vi "102_EON_presence_absence.vi"(8 "error in (no error)":errorcluster, 10 "Measurement ROI":T1 {"Contours"."Type" items=["No Selection", "Point", "Line", "Rectangle", "Oval", "Polygon", "Freehand Region", "Annulus", "Unused2", "Unused3", "Broken Line", "Freehand Line", "Rotated Rectangle"]}, 11 "Image In":T2(plugin-control)) -> (0 "error out":errorcluster, 2 "EON Presence/Absence":bool, 3 "Blob Center":cluster{"Center X":dbl, "Center Y":dbl})   [LabVIEW 2015]
uses:
  <vilib>/vision/NI_Vision_Development_Module.lvlib
  FrameworkOverrides/Algorithm.lvclass
panel:
  out "Area":dbl[](array[numeric])
  out "Area":dbl
  out "Y Coord":dbl[](array[numeric])
  out "Number of Particles":i32
  out "subarray 2":dbl[](array[numeric])
  out "index of element":i32
  out "Array":bool[](array[boolean])
  out "X Coord":dbl[](array[numeric])
  out "Image 2":T2(plugin-control)
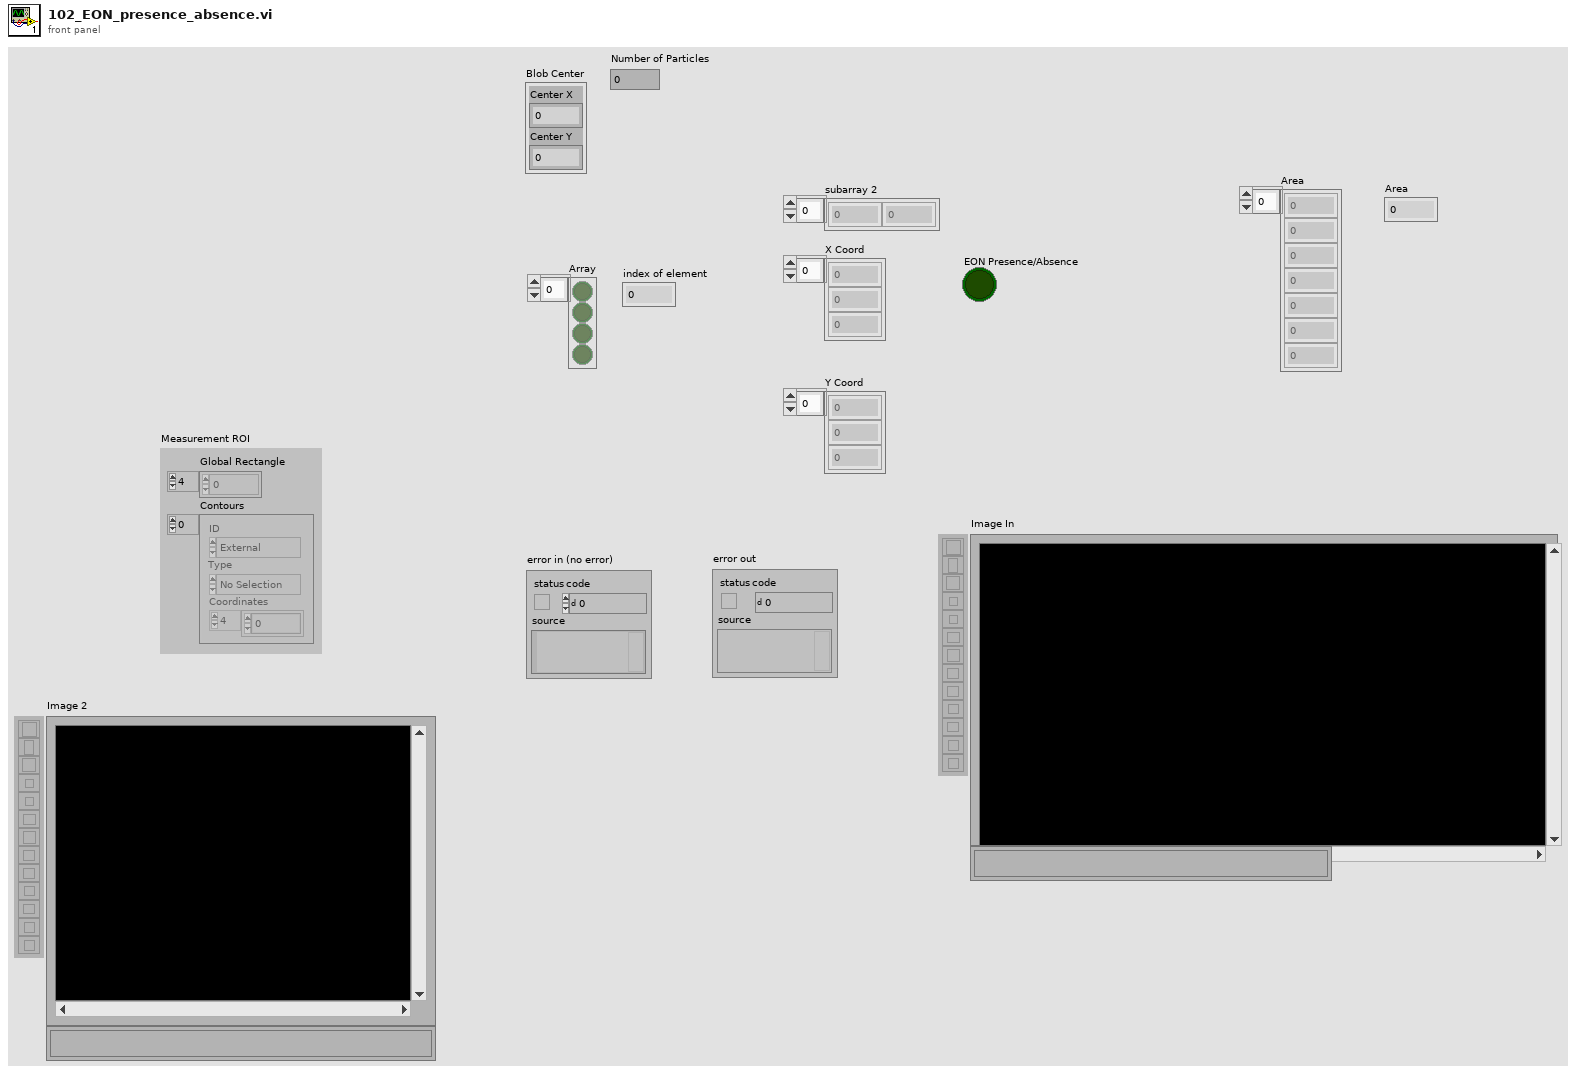
[diagram p1: front panel]
types:
  T1 = typedef "ROI Descriptor" = cluster{"Global Rectangle":i32[], "Contours":cluster{"ID":enum32{"External", "Internal"}, "Type":u32, "Coordinates":i32[]}[]}
  T2 = typedef "IMAQ Image.ctl" = refnum<image>
  T3 = typedef "Particle Parameters" = i32
  T4 = cluster{"Measurement Parameter":T3, "Range Lower Value":dbl, "Range Upper Value":dbl, "Range":bool, "Measurement Type":bool}[]
  T5 = typedef "Image Type" = u32
  T6 = typedef "IMAQ Rectangle" = cluster{"Left":i32, "Top":i32, "Right":i32, "Bottom":i32, "Rotation":dbl}
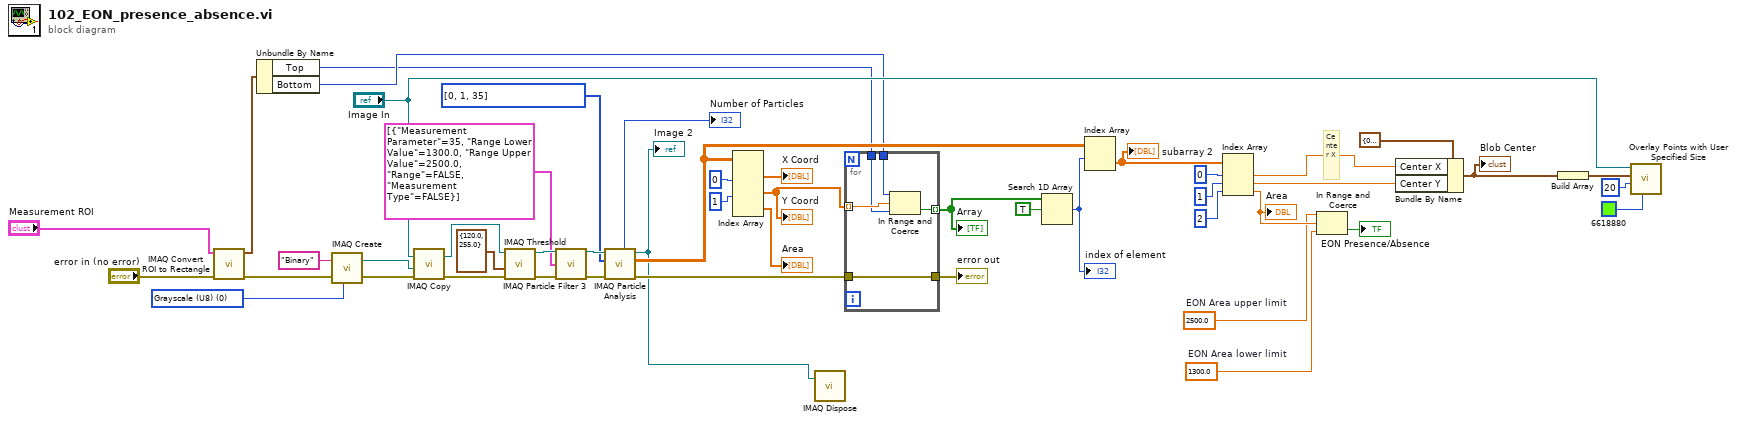
[diagram p0: block diagram]
diagram:
  w22 = 1300.0  # EON Area lower limit
  w23 = 2500.0  # EON Area upper limit
  w42 = T3[] [0, 1, 35] items=["Center of Mass X", "Center of Mass Y", "First Pixel X", "First Pixel Y", "Bounding Rect Left", "Bounding Rect Top", "Bounding Rect Right", "Bounding Rect Bottom", "Max Feret Diameter Start X", "Max Feret Diameter Start Y", "Max Feret Diameter End X", "Max Feret Diameter End Y", "Max Horiz. Segment Length Left", "Max Horiz. Segment Length Right", "Max Horiz. Segment Length Row", "-", "Bounding Rect Width", "Bounding Rect Height", "Bounding Rect Diagonal", "Perimeter", "Convex Hull Perimeter", "Holes' Perimeter", "Max Feret Diameter", "Equivalent Ellipse Major Axis", "Equivalent Ellipse Minor Axis", "Equivalent Ellipse Minor Axis (Feret)", "Equivalent Rect Long Side", "Equivalent Rect Short Side", "Equivalent Rect Diagonal", "Equivalent Rect Short Side (Feret)", "Average Horiz. Segment Length", "Average Vert. Segment Length", "Hydraulic Radius", "Waddel Disk Diameter", "-", "Area", "Holes' Area", "Particle & Holes' Area", "Convex Hull Area", "Image Area", "-", "Number of Holes", "Number of Horiz. Segments", "Number of Vert. Segments", "-", "Orientation", "Max Feret Diameter Orientation", "-", "% Area/Image Area", "% Area/(Particle & Holes' Area)", "Ratio of Equivalent Ellipse Axes", "Ratio of Equivalent Rect Sides", "-", "Elongation Factor", "Compactness Factor", "Heywood Circularity Factor", "Type Factor", "-", "Sum X", "Sum Y", "Sum XX", "Sum XY", "Sum YY", "Sum XXX", "Sum XXY", "Sum XYY", "Sum YYY", "-", "Moment of Inertia XX", "Moment of Inertia XY", "Moment of Inertia YY", "Moment of Inertia XXX", "Moment of Inertia XXY", "Moment of Inertia XYY", "Moment of Inertia YYY", "Norm. Moment of Inertia XX", "Norm. Moment of Inertia XY", "Norm. Moment of Inertia YY", "Norm. Moment of Inertia XXX", "Norm. Moment of Inertia XXY", "Norm. Moment of Inertia XYY", "Norm. Moment of Inertia YYY", "Hu Moment 1", "Hu Moment 2", "Hu Moment 3", "Hu Moment 4", "Hu Moment 5", "Hu Moment 6", "Hu Moment 7"] ("Pixel Measurements")
  w47 = T5 0 items=["Grayscale (U8)", "Grayscale (I16)", "Grayscale (SGL)", "Complex (CSG)", "RGB (U32)", "HSL (U32)", "RGB (U64)", "Grayscale (U16)"] ("Image Type")
  # "Center X"
  n1 = call "IMAQ Convert ROI to Rectangle"("error in (no error)"="error in (no error)", "ROI Descriptor"="Measurement ROI") -> ("error out"=w10:errorcluster, "Rectangle"=w11:T6)  [unwired: 7 in]
  n2 = Unbundle By Name(w11) -> ("Top"=w5:i32, "Bottom"=w6:i32)
  n3 = call "IMAQ Create"("Image Name"="Binary", "Image Type"=w47, "error in (no error)"=w10) -> ("New Image"=w1:T2, "error out"=w20:errorcluster)  [unwired: 2 in]
  n4 = call "IMAQ Copy"("error in (no error)"=w20, "Image Dst"=w1, "Image Src"="Image In") -> ("error out"=w26:errorcluster, "Image Dst Out"=w41:T2)  [unwired: 3 in]
  n5 = call "IMAQ Threshold"("error in (no error)"=w26, "Range"=cluster{"Lower value":sgl, "Upper value":sgl} {"Lower value"=120.0, "Upper value"=255.0}, "Image Src"=w41) -> ("error out"=w46:errorcluster, "Image Dst Out"=w45:T2)  [unwired: 7 in]
  n6 = call "IMAQ Particle Filter 3"("Image Src"=w45, "Selection Values"=T4 [{"Measurement Parameter"=35, "Range Lower Value"=1300.0, "Range Upper Value"=2500.0, "Range"=FALSE, "Measurement Type"=FALSE}], "error in (no error)"=w46) -> ("Image Dst Out"=w44:T2, "error out"=w43:errorcluster)  [unwired: 10 in, 1 out]
  n7 = call "IMAQ Particle Analysis"("error in (no error)"=w43, "Pixel Measurements"=w42, "Image"=w44) -> ("error out"=w8:errorcluster, "Particle Measurements (Pixels)"=w37:dbl[][], "Image Out (duplicate)"=w4:T2, "Number of Particles"=→"Number of Particles":i32)  [unwired: 3 in, 2 out]
  "Image 2" <- w4
  n8 = Index Array(array=w37, index (col) #1=0 ("disabled index (col)"), index (col) #2=1 ("index (col)")) -> (element #1=→"X Coord":dbl[], element #2=w29:dbl[], element #3=→"Area":dbl[])  [unwired: 4 in]
  "Y Coord" <- w29
  n9 = call "IMAQ Dispose"("Image"=w4) -> ()  [unwired: 5 in, 1 out]
  n10 = for {
    tunnel: w29 -> [w53] mode=indexing
    tunnel: [w52] -> w39 mode=indexing
    tunnel: w8 -> [w51]
    tunnel: [w51] -> w12
    tunnel: w6 -> [w50]
    tunnel: w5 -> [w49]
    n11 = In Range and Coerce(upper limit=w50, x=w53, lower limit=w49) -> (In Range?=w52:bool)  [unwired: 1 out]
  }
  "Array" <- w39
  "error out" <- w12
  n12 = Search 1D Array(1D array=w39, element=TRUE) -> (index of element=w36:i32)  [unwired: 1 in]
  "index of element" <- w36
  n13 = Index Array(array=w37, index (row)=w36) -> (element=w35:dbl[])  [unwired: 1 in]
  "subarray 2" <- w35
  n14 = Index Array(array=w35, index #1=0 ("index"), index #2=1 ("index"), index #3=2 ("index")) -> (element #1=w18:dbl, element #2=w17:dbl, element #3=w24:dbl)
  "Area" <- w24
  n15 = In Range and Coerce(upper limit=w23, x=w24, lower limit=w22) -> (In Range?=→"EON Presence/Absence":bool)  [unwired: 1 out]
  n16 = Bundle By Name(cluster=cluster{"Center X":dbl, "Center Y":dbl} {"Center X"=0.0, "Center Y"=0.0} ("Cluster"), "Center X"=w18, "Center Y"=w17) -> (w16:cluster{"Center X":dbl, "Center Y":dbl})
  "Blob Center" <- w16
  n17 = Build Array(w16) -> (w15:cluster{"Center X":dbl, "Center Y":dbl}[])
  n18 = call "Overlay Points with User Specified Size.vi"("Color"=u32 6618880, "Point Diameter (5)"=u32 20, "Points"=w15, "Image In"="Image In") -> ()  [unwired: 6 in, 2 out]
